vi "sub_TMtrans.vi"(10 "위도(lat)_Deg":dbl format="%#.6g", 11 "경도(lon)_Deg":dbl format="%#.6g") -> (2 "TM_Y(long)":dbl format="%#.6g", 3 "TM_X(lat)":dbl format="%#.6f")   [LabVIEW 2020]
uses:
  <vilib>/imath/engines/lvmath2/RunTimeEngine/Managers/WorkSpace/UID Generator.vi
  <vilib>/imath/engines/lvmath2/RunTimeEngine/RunTimeType/NIMS_RunTimeType_From StrictType (excl LVString).vi
  <instcachedir>/0/NIMS_RunTimeType_From StrictType (excl LVString)_283B1B2000484AAA8744D21CE97EA49F.lvgen/NIMS_RunTimeType_From StrictType (excl LVString)_283B1B2000484AAA8744D21CE97EA49F_000.vi
  <vilib>/imath/engines/lvmath2/RunTimeEngine/LocalVariableDefStatement/MC_LocalVariableDefStatement_Display.vi
  <vilib>/imath/engines/lvmath2/RunTimeEngine/Managers/SymbolTable/Clear UID.vi
  <vilib>/imath/engines/lvmath2/RunTimeEngine/NodeEndStatement/NIMS_NodeEndStatement_Output.vi
  <instcachedir>/0/NIMS_NodeEndStatement_Output_53EC0D466D134D7ABD903AC30B43404B.lvgen/NIMS_NodeEndStatement_Output_53EC0D466D134D7ABD903AC30B43404B_009.vi
  <vilib>/imath/engines/lvmath2/RunTimeEngine/ErrorHandling/NIMS_Finalize Error.vi
  <vilib>/imath/engines/lvmath2/RunTimeEngine/Managers/SymbolTable/NIMS_WorkSpace.lvlib
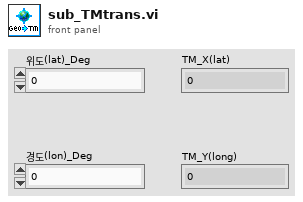
[diagram p1: front panel]
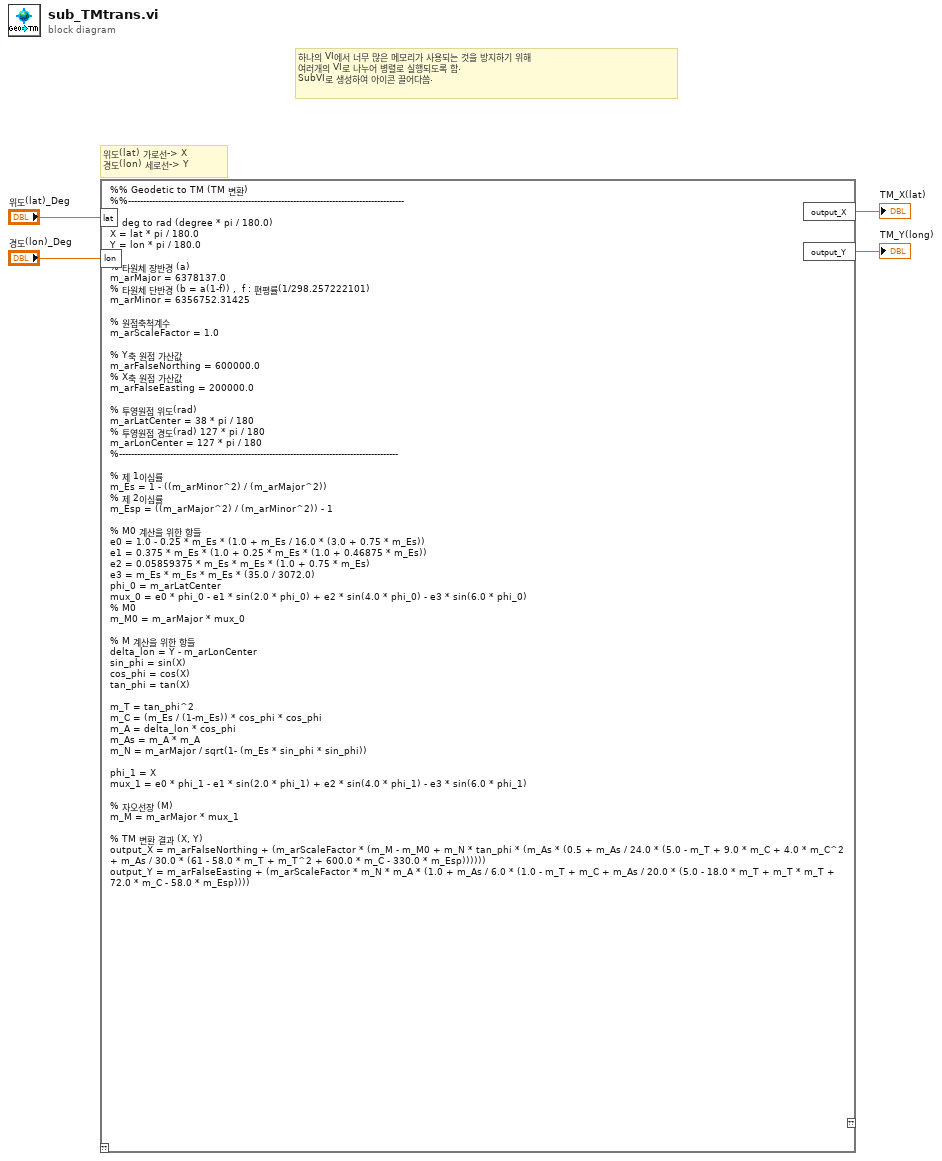
[diagram p0: block diagram]
diagram:
  # "위도(lat) 가로선-> X\n경도(lon) 세로선-> Y"
  # "하나의 VI에서 너무 많은 메모리가 사용되는 것을 방지하기 위해\n여러개의 VI로 나누어 병렬로 실행되도록 함.\nSubVI로 생성하여 아이콘 끌어다씀."
  n1 = mathscript code="%% Geodetic to TM (TM 변환)\n%%--------------------------------------------------------------------------------------------\n\n% deg to rad (degree * pi / 180.0)\nX = lat * pi / 180.0\nY = lon * pi / 180.0\n\n% 타원체 장반경 (a)\nm_arMajor = 6378137.0\n% 타원체 단반경 (b = a(1-f)) ,  f : 편평률(1/298.257222101)\nm_arMinor = 6356752.31425\n\n% 원점축척계수\nm_arScaleFactor = 1.0\n\n% Y축 원점 가산값 \nm_arFalseNorthing = 600000.0\n% X축 원점 가산값 \nm_arFalseEasting = 200000.0\n\n% 투영원점 위도(rad)\nm_arLatCenter = 38 * pi / 180\n% 투영원점 경도(rad) 127 * pi / 180\nm_arLonCenter = 127 * pi / 180\n%---------------------------------------------------------------------------------------------\n\n% 제 1이심률\nm_Es = 1 - ((m_arMinor^2) / (m_arMajor^2))\n% 제 2이심률\nm_Esp = ((m_arMajor^2) / (m_arMinor^2)) - 1\n\n% M0 계산을 위한 항들\ne0 = 1.0 - 0.25 * m_Es * (1.0 + m_Es / 16.0 * (3.0 + 0.75 * m_Es))\ne1 = 0.375 * m_Es * (1.0 + 0.25 * m_Es * (1.0 + 0.46875 * m_Es))\ne2 = 0.05859375 * m_Es * m_Es * (1.0 + 0.75 * m_Es)\ne3 = m_Es * m_Es * m_Es * (35.0 / 3072.0)\nphi_0 = m_arLatCenter\nmux_0 = e0 * phi_0 - e1 * sin(2.0 * phi_0) + e2 * sin(4.0 * phi_0) - e3 * sin(6.0 * phi_0)\n% M0\nm_M0 = m_arMajor * mux_0\n\n% M 계산을 위한 항들\ndelta_lon = Y - m_arLonCenter\nsin_phi = sin(X)\ncos_phi = cos(X)\ntan_phi = tan(X)\n\nm_T = tan_phi^2\nm_C = (m_Es / (1-m_Es)) * cos_phi * cos_phi\nm_A = delta_lon * cos_phi\nm_As = m_A * m_A\nm_N = m_arMajor / sqrt(1- (m_Es * sin_phi * sin_phi))\n\nphi_1 = X\nmux_1 = e0 * phi_1 - e1 * sin(2.0 * phi_1) + e2 * sin(4.0 * phi_1) - e3 * sin(6.0 * phi_1)\n\n% 자오선장 (M)\nm_M = m_arMajor * mux_1\n\n% TM 변환 결과 (X, Y)\noutput_X = m_arFalseNorthing + (m_arScaleFactor * (m_M - m_M0 + m_N * tan_phi * (m_As * (0.5 + m_As / 24.0 * (5.0 - m_T + 9.0 * m_C + 4.0 * m_C^2 + m_As / 30.0 * (61 - 58.0 * m_T + m_T^2 + 600.0 * m_C - 330.0 * m_Esp))))))\noutput_Y = m_arFalseEasting + (m_arScaleFactor * m_N * m_A * (1.0 + m_As / 6.0 * (1.0 - m_T + m_C + m_As / 20.0 * (5.0 - 18.0 * m_T + m_T * m_T + 72.0 * m_C - 58.0 * m_Esp))))"("lat"="위도(lat)_Deg", "lon"="경도(lon)_Deg") -> ("output_X"=→"TM_X(lat)":cdb, "output_Y"=→"TM_Y(long)":cdb)  [unwired: 1 in, 1 out]
